vi "Read Interactive.vi"(8 "error in (no error)":errorcluster, 11 "DefineSuite in":refnum<class "DestroySuite.lvclass">) -> (0 "error out":errorcluster, 2 "Interactive":bool, 3 "DefineSuite out":refnum<class "DestroySuite.lvclass">)   [LabVIEW 2021]
uses:
  DestroySuite.lvclass/DestroySuite.ctl
  DestroySuite.lvclass
  C:/Repositories/LVOS/Bananas/lv-src/Bananas/DestroySuite/DestroySuite.lvclass
  C:/Repositories/LVOS/Bananas/lv-src/Bananas/BananaPeel/BananaPeel.lvclass
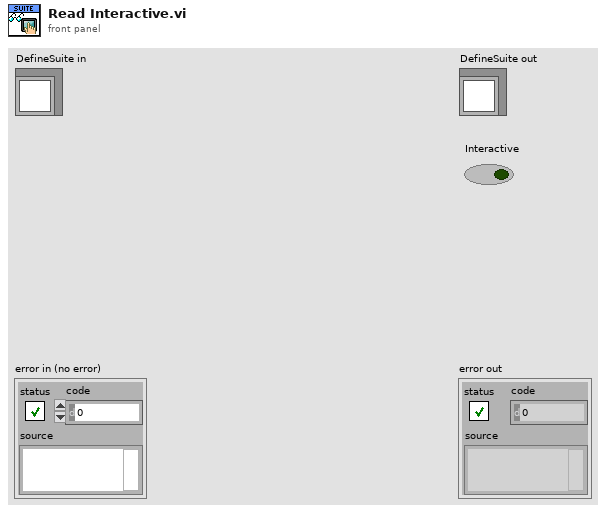
[diagram p1: front panel]
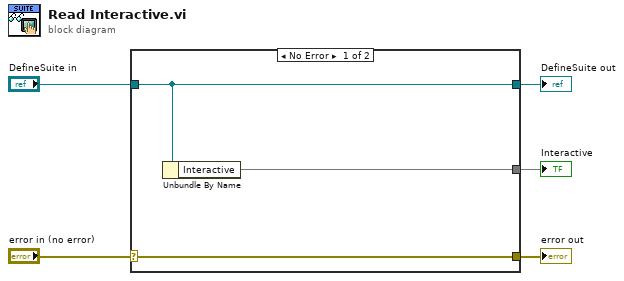
[diagram p0: block diagram]
diagram:
  n1 = case shown="No Error" "error in (no error)" {
    selector: "error in (no error)" -> [w8 w9]
    tunnel: [w8 w9] -> w4
    tunnel: [w7 w10] -> w2
    tunnel: "DefineSuite in" -> [w7 w10]
    tunnel: [w6 _] -> w1
    frame No Error {
      n2 = Unbundle By Name(w7) -> ("Interactive"=w6)
    }
    frame Error {
    }
  }
  "error out" <- w4
  "DefineSuite out" <- w2
  "Interactive" <- w1
